vi "Migrate 2_0_0.vi"(8 "error in (no error)":errorcluster, 10 "version":string, 11 "Device Ref in":T1 format="%.0x") -> (0 "error out":errorcluster, 2 "new version":string, 3 "Device Ref out":T1 format="%.0x")   [LabVIEW 2015, in "Chassis TimeSync System Explorer.lvlib"]
uses:
  Chassis TimeSync System Explorer.lvlib
  <vilib>/NI Veristand/Custom Device API/Custom Device Item Ref.ctl
  <vilib>/NI Veristand/Custom Device API/Custom Device Channel.ctl
  <vilib>/NI Veristand/Custom Device API/Custom Device Channel Type.ctl
  <vilib>/NI Veristand/Custom Device Tools/Custom Device Utility Library/Custom Device Utility Library.lvlib
  <vilib>/NI Veristand/Custom Device API/Custom Device API.lvlib
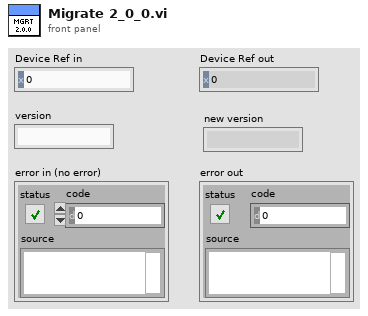
[diagram p1: front panel]
types:
  T1 = typedef "Custom Device API.lvlib/Custom Device Item Ref.ctl" = u64
  T2 = typedef "Custom Device API.lvlib/Custom Device Channel.ctl" = cluster{"Type":T3, "Units":string, "Default Value":dbl, "Faultable":bool, "Scalable":bool}
  T3 = typedef "Custom Device API.lvlib/Custom Device Channel Type.ctl" = enum16{"Input", "Output"}
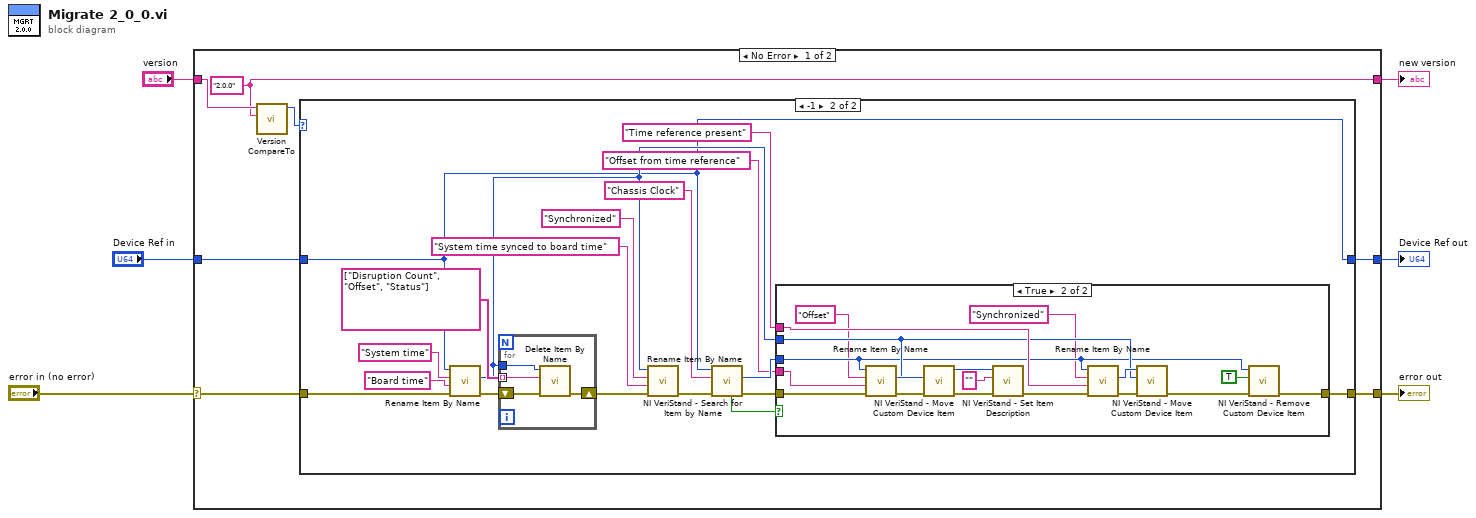
[diagram p0: block diagram]
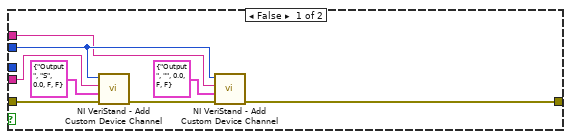
[diagram p3: hidden frame]
diagram:
  n1 = case shown="No Error" "error in (no error)" {
    selector: "error in (no error)" -> [w10 w66]
    tunnel: "version" -> [w12 w64]
    tunnel: [w11 w66] -> w5
    tunnel: "Device Ref in" -> [w9 w65]
    tunnel: [w8 w65] -> w2
    tunnel: [w7 w64] -> w1
    frame No Error {
      w7 = "2.0.0" ("version 2")
      n2 = call "Version CompareTo.vi"("version 2"=w7, "version 1"=w12) -> ("comparison"=w13:i32)  [unwired: 9 in]
      n3 = case shown="-1" w13 {
        tunnel: [w14 w16] -> w8
        tunnel: w9 -> [w14 w16]
        tunnel: w10 -> [w15 w31]
        tunnel: [w15 w18] -> w11
        frame Default {
          # "Already up to date"
        }
        frame -1 {
          n4 = call "Rename Item By Name.vi"("error in (no error)"=w31, "New Name"="Board time" ("Property Name"), "Old Name"="System time" ("Property Name"), "Parent Ref in"=w16) -> ("error out"=w30:errorcluster, "Item Ref out"=w17:T1)  [unwired: 5 in, 1 out]
          n5 = for {
            tunnel: string[] ["Disruption Count", "Offset", "Status"] ("Name") -> [w62] mode=indexing
            shift-right: [w61] -> w28
            shift-left: w30 -> [w63]
            tunnel: w17 -> [w60]
            n6 = call "Delete Item By Name.vi"("error in (no error)"=w63, "Name"=w62, "Parent Ref in"=w60) -> ("error out"=w61:errorcluster)  [unwired: 7 in, 1 out]
          }
          n7 = call "Rename Item By Name.vi"("error in (no error)"=w28, "New Name"="System time synced to board time", "Old Name"="Synchronized", "Parent Ref in"=w17) -> ("error out"=w24:errorcluster)  [unwired: 5 in, 2 out]
          n8 = call <vilib>:"NI VeriStand - Search for Item by Name.vi"("error in"=w24, "Item Name"="Chassis Clock", "Section Ref in"=w16) -> ("error out"=w22:errorcluster, "Item Ref"=w21:T1, "Found"=w23:bool)  [unwired: 5 in, 1 out]
          n9 = case shown="True" w23 {
            tunnel: w22 -> [w41 w59]
            tunnel: w21 -> [_ w49]
            tunnel: w17 -> [w37 w53]
            tunnel: "Time reference present" ("New Name") -> [w36 w56]
            tunnel: "Offset from time reference" ("New Name") -> [w40 w55]
            tunnel: [w38 w50] -> w18
            frame False {
              n10 = call <vilib>:"NI VeriStand - Add Custom Device Channel.vi"("error in (no error)"=w41, "Channel"=T2 {"Type"=enum."Output", "Units"="S", "Default Value"=0.0, "Faultable"=FALSE, "Scalable"=FALSE}, "Channel Name"=w40, "Parent Ref in"=w37) -> ("error out"=w39:errorcluster)  [unwired: 4 in, 3 out]
              n11 = call <vilib>:"NI VeriStand - Add Custom Device Channel.vi"("error in (no error)"=w39, "Channel"=T2 {"Type"=enum."Output", "Units"="", "Default Value"=0.0, "Faultable"=FALSE, "Scalable"=FALSE}, "Channel Name"=w36, "Parent Ref in"=w37) -> ("error out"=w38:errorcluster)  [unwired: 4 in, 3 out]
            }
            frame True {
              n12 = call "Rename Item By Name.vi"("error in (no error)"=w59, "New Name"=w55, "Old Name"="Offset", "Parent Ref in"=w49) -> ("error out"=w58:errorcluster, "Item Ref out"=w57:T1)  [unwired: 5 in, 1 out]
              n13 = call <vilib>:"NI VeriStand - Move Custom Device Item.vi"("error in (no error)"=w58, "New Parent Ref in"=w53, "Item Ref in"=w57) -> ("error out"=w46:errorcluster, "Item Ref out"=w44:T1)  [unwired: 6 in, 1 out]
              n14 = call <vilib>:"NI VeriStand - Set Item Description.vi"("error in (no error)"=w46, "Description"="", "Item Ref in"=w44) -> ("error out"=w45:errorcluster)  [unwired: 6 in, 2 out]
              n15 = call "Rename Item By Name.vi"("error in (no error)"=w45, "New Name"=w56, "Old Name"="Synchronized", "Parent Ref in"=w49) -> ("error out"=w52:errorcluster, "Item Ref out"=w54:T1)  [unwired: 5 in, 1 out]
              n16 = call <vilib>:"NI VeriStand - Move Custom Device Item.vi"("error in (no error)"=w52, "New Parent Ref in"=w53, "Item Ref in"=w54) -> ("error out"=w42:errorcluster)  [unwired: 6 in, 2 out]
              n17 = call <vilib>:"NI VeriStand - Remove Custom Device Item.vi"("error in (no error)"=w42, "Force Delete (F)"=TRUE, "Item Ref in"=w49) -> ("error out"=w50:errorcluster)  [unwired: 7 in, 1 out]
            }
          }
        }
      }
    }
    frame Error {
    }
  }
  "error out" <- w5
  "Device Ref out" <- w2
  "new version" <- w1
